vi "GetCallerLibraryName.vi"(8 "error in (no error)":errorcluster) -> (0 "error out":errorcluster, 3 "Name":string)   [LabVIEW 2017, in "Communication.lvlib"]
uses:
  Communication.lvlib
  <vilib>/Utility/error.llb/Error Cluster From Error Code.vi
  <vilib>/ErrorRing/Error Ring.xnode
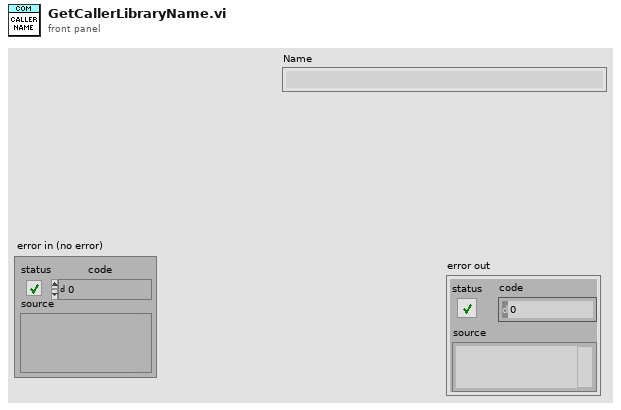
[diagram p1: front panel]
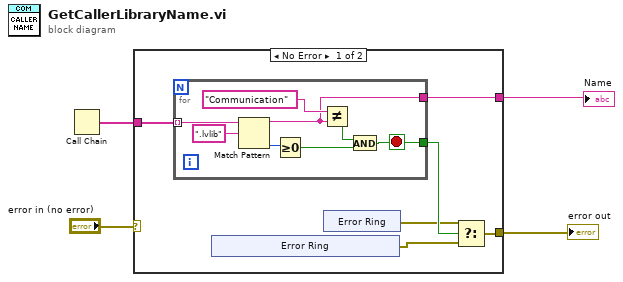
[diagram p0: block diagram]
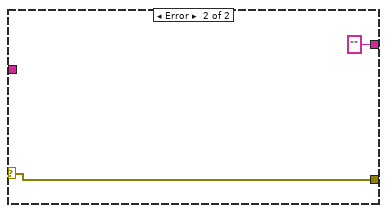
[diagram p2: hidden frame]
diagram:
  n1 = Call Chain() -> (call chain=w4:string[])
  n2 = case shown="No Error" "error in (no error)" {
    selector: "error in (no error)" -> [_ w26]
    tunnel: w4 -> [w10 _]
    tunnel: [w9 ""] -> w3
    tunnel: [w6 w26] -> w1
    frame No Error {
      n3 = for {
        tunnel: w10 -> [w23] mode=indexing
        tunnel: [w18] -> w9
        tunnel: [w17] -> w7
        stop <- w17 stop-if-true
        n4 = Match Pattern(string=w23, regular expression=".lvlib") -> (before substring=w18:string, offset past match=w22:i32)  [unwired: 1 in, 2 out]
        n5 = Greater Or Equal To 0?(x=w22) -> (x >= 0?=w19:bool)
        n6 = Not Equal?(x="Communication", y=w18) -> (x != y?=w20:bool)
        n7 = And(x=w20, y=w19) -> (x .and. y?=w17:bool)
      }
      n8 = xnode "Error Ring"() -> ("error out"=w8:errorcluster)
      n9 = xnode "Error Ring"() -> ("error out"=w5:errorcluster)
      n10 = Select(t=w5, s=w7, f=w8) -> (s? t:f=w6:errorcluster)
    }
    frame Error {
    }
  }
  "Name" <- w3
  "error out" <- w1
